vi "SetGageConfig_SW.vi"(0 "Handle Cluster":T4, 1 "Slope":refnum<vi>, 2 "External Coupling":refnum<vi>, 3 "Mode":refnum<vi>, 5 "Channels":T1(array[cluster]), 9 "Acquisition":T2, 11 "Trigger":T3, 12 "Coupling":refnum<vi>, 13 "External Inpedance":refnum<vi>) -> ()   [LabVIEW 2013]
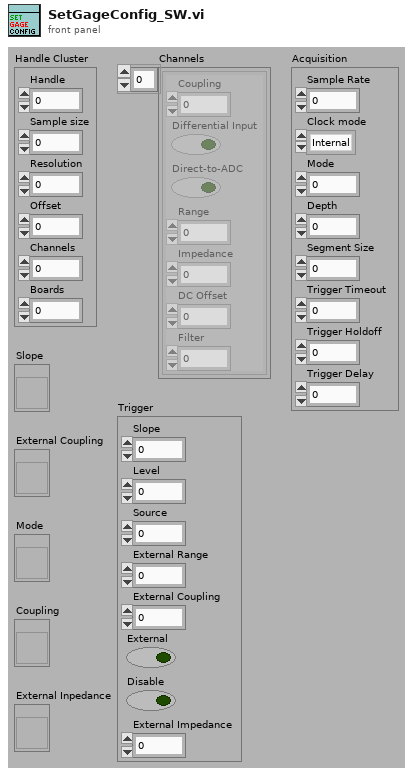
[diagram p1: front panel]
types:
  T1 = cluster{"Coupling":u16, "Differential Input":bool, "Direct-to-ADC":bool, "Range":u32, "Impedance":u32, "DC Offset":i32, "Filter":i32}[]
  T2 = cluster{"Sample Rate":dbl, "Clock mode":enum16{"Internal", "External", "Reference"}, "Mode":u16, "Depth":dbl, "Segment Size":dbl, "Trigger Timeout":dbl, "Trigger Holdoff":dbl, "Trigger Delay":dbl}
  T3 = cluster{"Slope":u16, "Level":i32, "Source":i32, "External Range":u32, "External Coupling":u16, "External":bool, "Disable":bool, "External Impedance":u16}
  T4 = cluster{"Handle":u32, "Sample size":u32, "Resolution":i32, "Offset":i32, "Channels":u32, "Boards":u32}
  T5 = cluster{string, "Differential Input":bool, "Direct-to-ADC":bool, "Range":u32, "Impedance":u32, "DC Offset":i32, u32}
  T6 = cluster{"RingText.Text":string, "Level":i32, "Source":i32, "External Range":u32, "RingText.Text":string, "External":bool, "Disable":bool, "RingText.Text":string}
  T7 = cluster{"RingText.Text":string, "Level":i32, "Source":i32, "External Range":u32, "RingText.Text":string, "External":bool, "Disable":bool, "RingText.Text":string}[]
  T8 = cluster{"Sample Rate":dbl, "Clock mode":enum16{"Internal", "External", "Reference"}, "RingText.Text":string, "Depth":dbl, "Segment Size":dbl, "Trigger Timeout":dbl, "Trigger Holdoff":dbl, "Trigger Delay":dbl}
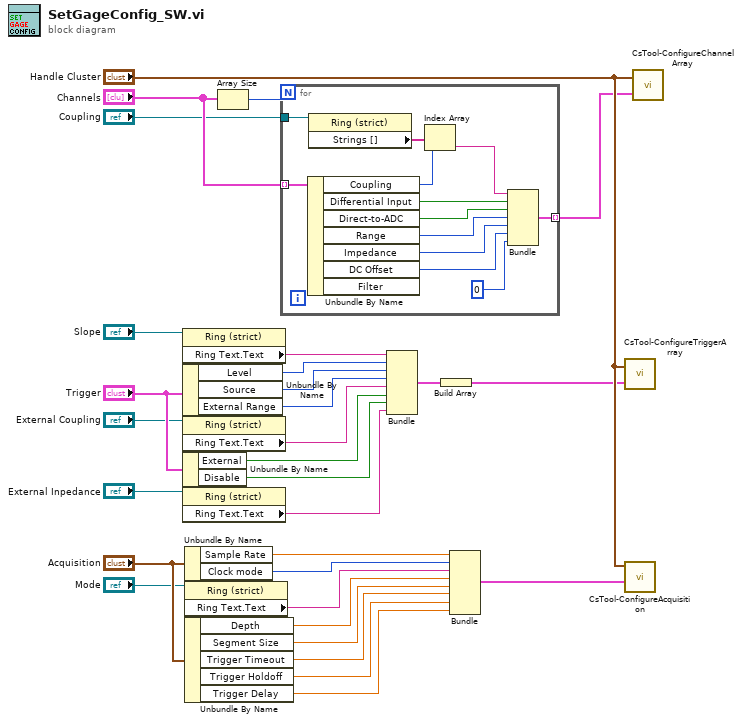
[diagram p0: block diagram]
diagram:
  n1 = property on="Property Node" class="Ring (strict)"(reference="Slope") -> ("Ring Text.Text"=w7:string)  [unwired: 1 in, 2 out]
  n2 = Unbundle By Name("Trigger") -> ("Level"=w8:i32, "Source"=w26:i32, "External Range"=w27:u32)
  n3 = property on="Property Node" class="Ring (strict)"(reference="External Coupling") -> ("Ring Text.Text"=w9:string)  [unwired: 1 in, 2 out]
  n4 = Unbundle By Name("Trigger") -> ("External"=w19:bool, "Disable"=w28:bool)
  n5 = property on="Property Node" class="Ring (strict)"(reference="External Inpedance") -> ("Ring Text.Text"=w29:string)  [unwired: 1 in, 2 out]
  n6 = Unbundle By Name("Acquisition") -> ("Sample Rate"=w11:dbl, "Clock mode"=w20:enum16{"Internal", "External", "Reference"})
  n7 = property on="Property Node" class="Ring (strict)"(reference="Mode") -> ("Ring Text.Text"=w12:string)  [unwired: 1 in, 2 out]
  n8 = Unbundle By Name("Acquisition") -> ("Depth"=w13:dbl, "Segment Size"=w21:dbl, "Trigger Timeout"=w22:dbl, "Trigger Holdoff"=w23:dbl, "Trigger Delay"=w24:dbl)
  n9 = Array Size(array="Channels") -> (size(s)=w15:i32)
  n10 = for {
    N: w15 -> [_]
    tunnel: "Channels" -> [w40] mode=indexing
    tunnel: [w41] -> w1 mode=indexing
    tunnel: "Coupling" -> [w31]
    n11 = Unbundle By Name(w40) -> ("Coupling"=w36:u16, "Differential Input"=w42:bool, "Direct-to-ADC"=w35:bool, "Range"=w34:u32, "Impedance"=w33:u32, "DC Offset"=w32:i32)  [unwired: 1 out]
    n12 = property on="Property Node" class="Ring (strict)"(reference=w31) -> ("Strings []"=w39:string[])  [unwired: 1 in, 2 out]
    n13 = Index Array(array=w39, index=w36) -> (element=w38:string)
    n14 = Bundle(w38, "Differential Input"=w42, "Direct-to-ADC"=w35, "Range"=w34, "Impedance"=w33, "DC Offset"=w32, u32 0) -> (w41:T5)  [unwired: 1 in]
  }
  n15 = Bundle("RingText.Text"=w7, "Level"=w8, "Source"=w26, "External Range"=w27, "RingText.Text"=w9, "External"=w19, "Disable"=w28, "RingText.Text"=w29) -> (w10:T6)  [unwired: 1 in]
  n16 = Build Array(w10) -> (w17:T7)
  n17 = Bundle("Sample Rate"=w11, "Clock mode"=w20, "RingText.Text"=w12, "Depth"=w13, "Segment Size"=w21, "Trigger Timeout"=w22, "Trigger Holdoff"=w23, "Trigger Delay"=w24) -> (w25:T8)  [unwired: 1 in]
  n18 = call <instrlib>:"CsTool-ConfigureTriggerArray.vi"("Triggers"=w17, "Handle Cluster"="Handle Cluster") -> ()  [unwired: 1 out]
  n19 = call <instrlib>:"CsTool-ConfigureAcquisition.vi"("Acquisition"=w25, "Handle Cluster"="Handle Cluster") -> ()  [unwired: 9 in, 1 out]
  n20 = call <instrlib>:"CsTool-ConfigureChannelArray.vi"("Channels"=w1, "Handle Cluster"="Handle Cluster") -> ()  [unwired: 1 out]
